vi "Store ILC Data.vi"(8 "error in (no error)":errorcluster, 11 "Model in":refnum<class "Model.lvclass">) -> (0 "error out":errorcluster, 3 "Model out":refnum<class "Model.lvclass">)   [LabVIEW 2016, in "Model.lvclass"]
uses:
  Model.lvclass
  Model.lvclass/Model.ctl
  common_rt_hpilc/HPILC/HPILC.lvclass/HPILC.ctl
  common_rt_hpilc/HPILC/HPILC.lvclass
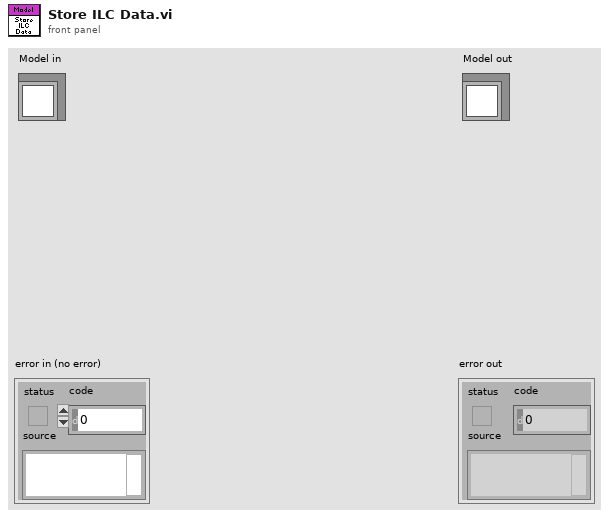
[diagram p1: front panel]
types:
  T1 = typedef "HPMT_Typedefs.lvlib/ActuatorData.ctl" = cluster{"Timestamp":dbl, "Force":dbl, "Encoder Value":i32, "Displacement Sensor 1":dbl, "Displacement Sensor 2":dbl, "Limit Switch CW":bool, "Limit Switch CCW":bool}
  T2 = typedef "RTHPILC.lvlib/HPData.ctl" = cluster{"Constants":T3, "Command":T4, "Telemetry":T5, "Responses":T6, "Timings":T8}
  T3 = typedef "RTHPILC.lvlib/HPConstants.ctl" = cluster{"ID":i16, "ReferencePosition":i32}
  T4 = typedef "RTHPILC.lvlib/HPCommand.ctl" = cluster{"Steps":i8}
  T5 = typedef "RTHPILC.lvlib/HPTelemetry.ctl" = cluster{"ILCFault":bool, "LimitSwitchCWOperated":bool, "LimitSwitchCCWOperated":bool, "BroadcastCounter":u8, "SSIEncoderValue":i32, "LoadCellForce":sgl}
  T6 = typedef "RTHPILC.lvlib/HPResponses.ctl" = cluster{"StepMotor":T7, "ForceAndStatus":T7}
  T7 = typedef "RTModbus.lvlib/ExceptionCodes.ctl" = u16
  T8 = typedef "RTHPILC.lvlib/HPTimings.ctl" = cluster{"BroadcastStepMotor":u32, "ForceAndStatus":u32, "FreezeSensorValues":u32, "StepMotor":u32}
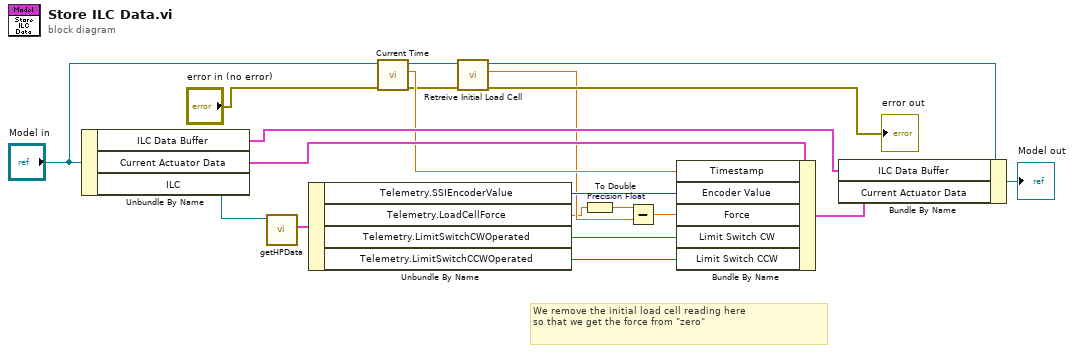
[diagram p0: block diagram]
diagram:
  # "We remove the initial load cell reading here\nso that we get the force from \"zero\""
  n1 = Unbundle By Name("Model in") -> ("ILC Data Buffer"=w20:T1[], "Current Actuator Data"=w19:T1, "ILC"=w18:refnum<class "HPILC.lvclass">)
  n2 = call "getHPData.vi"("HPILC in"=w18) -> ("HPData"=w17:T2)  [unwired: 9 in, 1 out]
  n3 = Unbundle By Name(w17) -> ("Telemetry.SSIEncoderValue"=w16:i32, "Telemetry.LoadCellForce"=w1:sgl, "Telemetry.LimitSwitchCWOperated"=w14:bool, "Telemetry.LimitSwitchCCWOperated"=w13:bool)
  n4 = call "Current Time.vi"("error in (no error)"="error in (no error)", "Model in"="Model in") -> ("error out"=w6:errorcluster, "Time"=w8:dbl, "Model out"=w11:refnum<class "Model.lvclass">)  [unwired: 7 in]
  n5 = call-dynamic "Retreive Initial Load Cell.vi"("error in (no error)"=w6, "Model in"=w11) -> ("error out"=→"error out":errorcluster, "Load Cell Reading"=w3:dbl, "Model out"=w7:refnum<class "Model.lvclass">)  [unwired: 7 in]
  n6 = To Double Precision Float(number=w1) -> (double precision float=w2:dbl)
  n7 = Subtract(x=w2, y=w3) -> (x-y=w4:dbl)
  n8 = Bundle By Name(cluster=w19, "Timestamp"=w8, "Encoder Value"=w16, "Force"=w4, "Limit Switch CW"=w14, "Limit Switch CCW"=w13) -> (w15:T1)
  n9 = Bundle By Name(cluster=w7, "ILC Data Buffer"=w20, "Current Actuator Data"=w15) -> (→"Model out":refnum<class "Model.lvclass">)
